vi "FGV_PlotStyle_ConvLineColor.vi"(3 "spreadsheet string":string, 4 "LineColorArray":u32[](array[numeric]), 5 "Func":enum16{"Write", "Read"}(ring)) -> (0 "spreadsheet string":string, 1 "LineColorArray":u32[](array[numeric]))   [LabVIEW 2018]
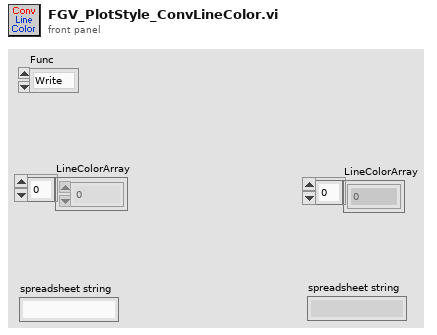
[diagram p1: front panel]
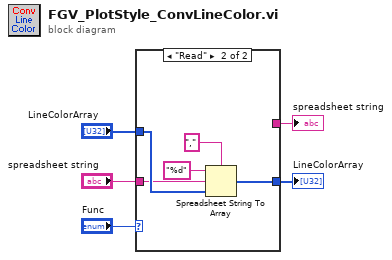
[diagram p0: block diagram]
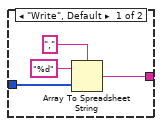
[diagram p2: hidden frame]
diagram:
  n1 = case shown="\"Read\"" "Func" {
    tunnel: "LineColorArray" -> [w7 w14]
    tunnel: [w6 _] -> w3
    tunnel: "spreadsheet string" -> [_ w13]
    tunnel: [_ w10] -> w1
    frame "Write", Default {
      n2 = Array To Spreadsheet String(delimiter (Tab)=",", array=w7, 3:"%d" ("format string")) -> (spreadsheet string=w6:string)
    }
    frame "Read" {
      n3 = Spreadsheet String To Array(delimiter (Tab)=",", format string="%d", spreadsheet string=w13, array type (2D Dbl)=w14) -> (array=w10:u32[])
    }
  }
  "spreadsheet string" <- w3
  "LineColorArray" <- w1
